vi "test13.vi"   [LabVIEW 2012]
uses:
  <vilib>/NXT/Subs/MotorOutput.ctl
  <vilib>/NXT/Dual Mode Library/Motors/MotorReverse.vi
  <vilib>/NXT/Dual Mode Library/Motors/MotorBrake.vi
  <vilib>/NXT/Dual Mode Library/Waits/Wait_Num(msec).vi
types:
  T1 = typedef "LVHSConnector.ctl" = cluster{"Hardware":string, "Flattened String":string}
  T2 = typedef "MotorOutput.ctl" = u8
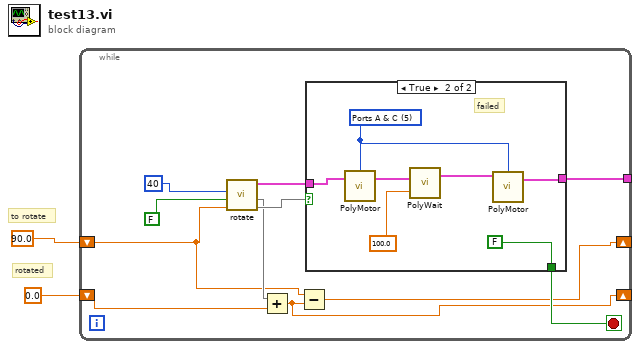
[diagram p0: block diagram]
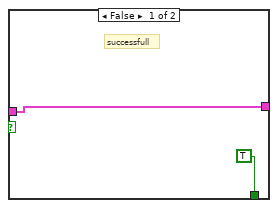
[diagram p2: hidden frame]
diagram:
  # "rotated"
  # "to rotate"
  n1 = while {
    shift-right: [w5] -> _
    shift-left: 90.0 ("degrees to  rotate") -> [w6]
    shift-right: [w4] -> _
    shift-left: 0.0 ("degrees to  rotate") -> [w8]
    tunnel: [w3] -> _
    stop <- w10 stop-if-true
    n2 = call "rotate.vi"("degrees to  rotate"=w6, "right(T)/left(F)"=FALSE, "power"=u16 40) -> (0:w13, 1:w7, "NXT"=w9:T1)  [unwired: 6 in]
    n3 = Add(x=w7, y=w8) -> (x+y=w4:dbl)
    n4 = Subtract(x=w6, y=w4) -> (x-y=w5:dbl)
    n5 = case shown="True" w13 {
      tunnel: [TRUE FALSE] -> w10
      tunnel: w9 -> [w14 w21]
      tunnel: [w14 w16] -> w3
      frame False {
        # "successfull"
      }
      frame True {
        w18 = T2 5 items=["Port A"=0, "Port B"=1, "Port C"=2, "Ports A & B"=4, "Ports A & C"=5, "Ports B & C"=6, "All Ports"=3] ("Output Port (All Ports)")
        # "failed"
        n6 = call-poly <vilib>:"PolyMotor.vi"("NXT"=w21, "Output Port (All Ports)"=w18) -> ("NXT"=w17:T1)  [unwired: 2 in]
        n7 = call-poly <vilib>:"PolyWait.vi"("Time (100 msec)"=sgl 100.0 ("Time (1 sec)"), "NXT"=w17) -> ("NXT"=w19:T1)  [unwired: 2 in]
        n8 = call-poly <vilib>:"PolyMotor.vi"("NXT"=w19, "Port (All Ports)"=w18) -> ("NXT"=w16:T1)  [unwired: 2 in]
      }
    }
  }
